vi "Get Distance.vi"(6 "distance/rotation":dbl=24.37875899 format="%#_13g", 10 "Starting value":dbl, 11 "PotDevRef":T1) -> (3 "Distance":dbl)   [LabVIEW 2017]
uses:
  <vilib>/Rock Robotics/WPI/Potentiometer/WPI_PotentiometerDevRef.ctl
  <vilib>/Rock Robotics/SystemInterfaces/AI/FPGA_AIChannel.ctl
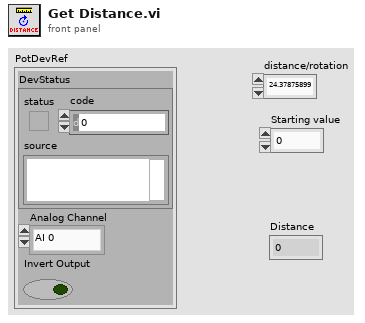
[diagram p1: front panel]
types:
  T1 = typedef "WPI_PotentiometerDevRef.ctl" = cluster{"DevStatus":errorcluster, "Analog Channel":T2, "Invert Output":bool}
  T2 = typedef "FPGA_AIChannel.ctl" = enum8{"AI 0", "AI 1", "AI 2", "AI 3", "AI MXP 0", "AI MXP 1", "AI MXP 2", "AI MXP 3", "Invalid"}
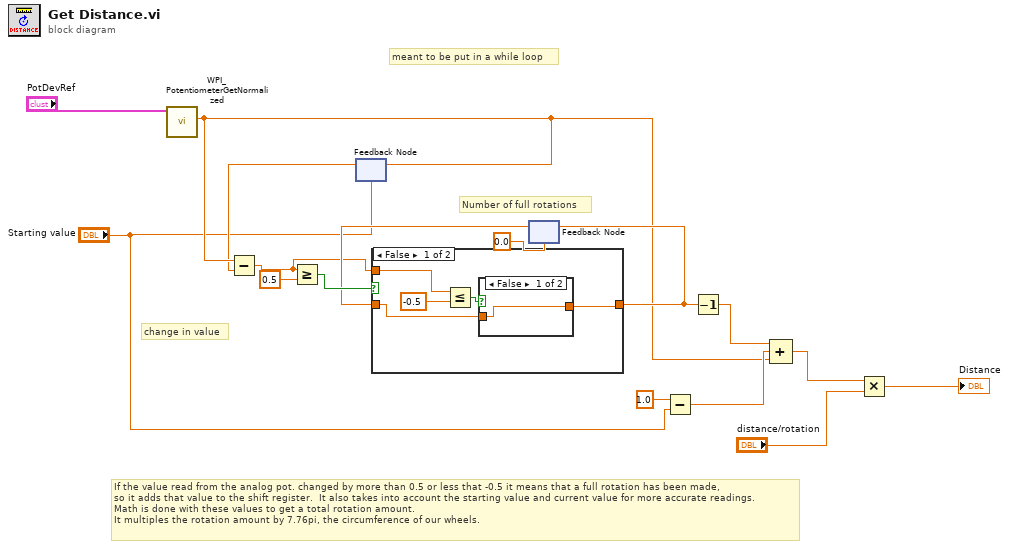
[diagram p0: block diagram]
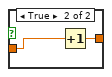
[diagram p2: hidden frame]
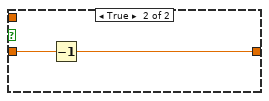
[diagram p3: hidden frame]
diagram:
  # "meant to be put in a while loop"
  # "change in value"
  # "Number of full rotations"
  # "If the value read from the analog pot. changed by more than 0.5 or less that -0.5 it means that a full rotation has been made, \nso it adds that value to the shift register.  It also takes into account the starting value and current value for more accurate readings.\nMath is done with these values to get a total rotation amount.\nIt multiples the rotation amount by 7.76pi, the circumference of our wheels."
  n1 = call <vilib>:"WPI_PotentiometerGetNormalized.vi"("PotDevRef"="PotDevRef") -> ("Normalized Value"=w6:dbl)  [unwired: 8 in, 2 out]
  n2 = feedback #1("Starting value") -> (w5:dbl)
  n3 = Subtract(x=w6, y=w5) -> (x-y=w11:dbl)
  n4 = Greater Or Equal?(x=w11, y=0.5) -> (x >= y?=w13:bool)
  n5 = feedback-in #1(w6) -> ()
  n6 = feedback #2(0.0) -> (w12:dbl)
  n7 = case shown="False" w13 {
    tunnel: [w17 w26] -> w9
    tunnel: w12 -> [w18 w25]
    tunnel: w11 -> [w21 _]
    frame False {
      n8 = Less Or Equal?(x=w21, y=-0.5) -> (x <= y?=w19:bool)
      n9 = case shown="False" w19 {
        tunnel: w18 -> [w22 w24]
        tunnel: [w22 w23] -> w17
        frame False {
        }
        frame True {
          n10 = Increment(x=w24) -> (x+1=w23:dbl)
        }
      }
    }
    frame True {
      n11 = Decrement(x=w25) -> (x-1=w26:dbl)
    }
  }
  n12 = feedback-in #2(w9) -> ()
  n13 = Subtract(x=1.0, y="Starting value") -> (x-y=w7:dbl)
  n14 = Decrement(x=w9) -> (x-1=w8:dbl)
  n15 = Compound Arithmetic op=ADD(w8, w7, w6) -> (w1:dbl)
  n16 = Multiply(x=w1, y="distance/rotation") -> (x*y=→"Distance":dbl)
